vi "NI.History (EXT).vi"(1 "value in":ext) -> (0 "Stop?":bool)   [LabVIEW 2020]
doc: "Displays the value of the 32-bit signed integer numeric control and allows conditional breakpoints."
uses:
  <vilib>/Utility/miscctls.llb/LVRowAndColumnUnsignedTypeDef.ctl
panel:
  out "History":i32(listbox)=-1
  in  "Format":string="%#_g"
  in  "reset":bool
  # "* Changes to these options take effect the next time the probe runs."
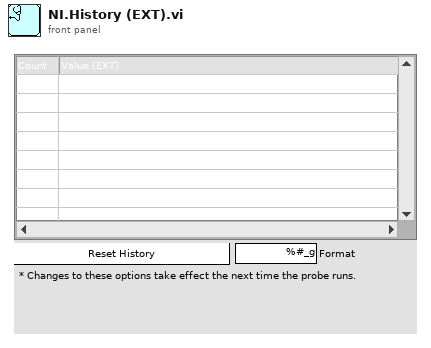
[diagram p1: front panel]
types:
  T1 = typedef "LVRowAndColumnUnsignedTypeDef.ctl" = cluster{"Row":u32, "Column":u32}
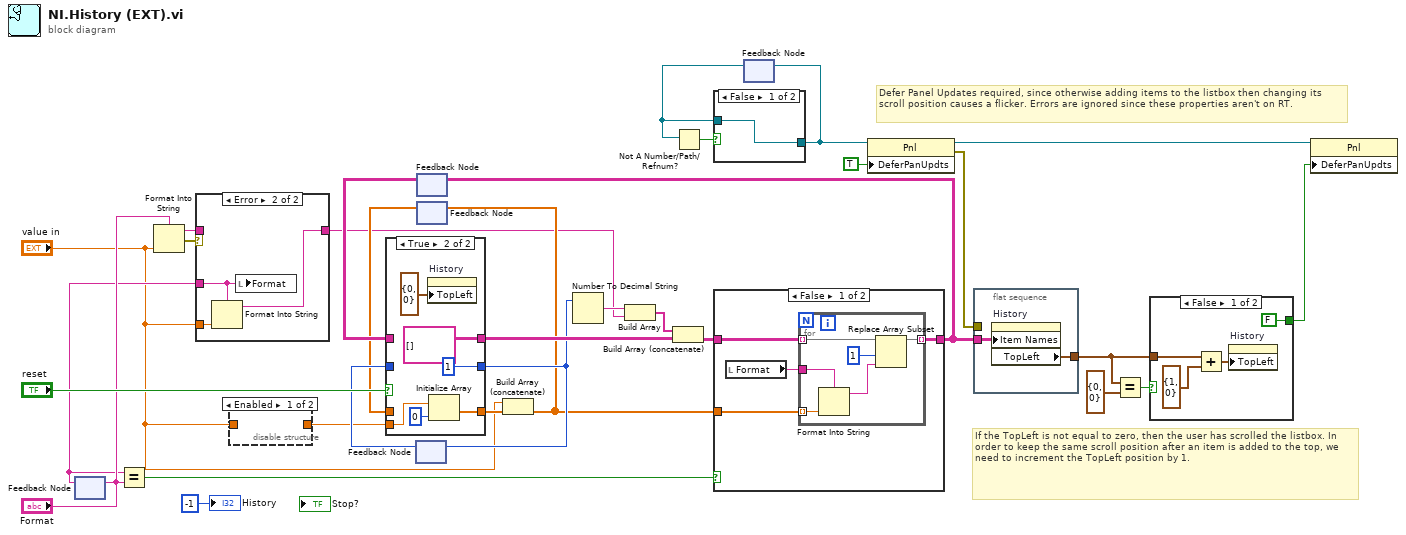
[diagram p0: block diagram]
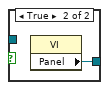
[diagram p3: hidden frame]
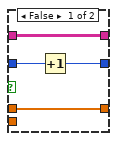
[diagram p6: hidden frame]
diagram:
  # "If the TopLeft is not equal to zero, then the user has scrolled the listbox. In order to keep the same scroll position after an item is added to the top, we need to increment the TopLeft position by 1."
  # "Defer Panel Updates required, since otherwise adding items to the listbox then changing its scroll position causes a flicker. Errors are ignored since these properties aren't on RT."
  n1 = feedback #1() -> (w15:string)  [unwired: 1 in]
  n2 = feedback-in #1("Format") -> ()
  n3 = Equal?(x=w15, y="Format") -> (x = y?=w17:bool)
  n4 = Format Into String(format string="Format", "value in") -> (resulting string=w12:string, error out=w13:errorcluster)  [unwired: 2 in]
  n5 = case shown="Error" w13 {
    tunnel: w15 -> [_ w34]
    tunnel: w12 -> [w32 _]
    tunnel: [w32 w33] -> w14
    tunnel: "value in" -> [_ w35]
    frame No Error {
    }
    frame Error {
      n6 = Format Into String(format string=w34, w35) -> (resulting string=w33:string)  [unwired: 2 in, 1 out]
      n7 = local write "Format"(w34) -> ()
    }
  }
  n8 = disable-structure shown="Enabled" {
    disable-tunnel: "value in" -> [_ w36]
    disable-tunnel: [_ w36] -> w21
    frame Enabled {
    }
    frame Disabled {
    }
  }
  n9 = feedback #2() -> (w25:i32)  [unwired: 1 in]
  n10 = feedback #3() -> (w24:string[][])  [unwired: 1 in]
  n11 = feedback #4() -> (w19:ext[])  [unwired: 1 in]
  n12 = case shown="True" "reset" {
    tunnel: w24 -> [w40 _]
    tunnel: w25 -> [w39 _]
    tunnel: [w40 string[][] []] -> w29
    tunnel: [w38 1] -> w26
    tunnel: w21 -> [_ w44]
    tunnel: [w37 w42] -> w20
    tunnel: w19 -> [w37 _]
    frame False {
      n13 = Increment(x=w39) -> (x+1=w38:i32)
    }
    frame True {
      n14 = property on="History" class="MCListbox (strict)"("TopLeft"=T1 {"Row"=0, "Column"=0} ("Top Left Visible Cell")) -> ()  [unwired: 2 in, 2 out]
      n15 = Initialize Array(w44, 0 ("dimension size")) -> (w42:ext[])
    }
  }
  n16 = feedback-in #2(w26) -> ()
  n17 = Build Array (concatenate)("value in", w20) -> (w18:ext[])
  n18 = feedback-in #4(w18) -> ()
  n19 = Number To Decimal String(number=w26) -> (decimal integer string=w27:string)  [unwired: 1 in]
  n20 = Build Array(w27, w14) -> (w28:string[])
  n21 = Build Array (concatenate)(w28, w29) -> (w22:string[][])
  n22 = case shown="False" w17 {
    tunnel: [w49 w57] -> w23
    tunnel: w22 -> [w50 w57]
    tunnel: w18 -> [w48 _]
    frame False {
      n23 = local read "Format"() -> (w47:string)
      n24 = for {
        tunnel: w50 -> [w56] mode=indexing
        tunnel: [w55] -> w49 mode=indexing
        tunnel: w48 -> [w53] mode=indexing
        tunnel: w47 -> [w51]
        n25 = Format Into String(format string=w51, w53) -> (resulting string=w52:string)  [unwired: 2 in, 1 out]
        n26 = Replace Array Subset(array=w56, new element=w52, index=1) -> (w55:string[])
      }
    }
    frame True {
    }
  }
  n27 = feedback-in #3(w23) -> ()
  n28 = feedback #5() -> (w7:refnum<vi>)  [unwired: 1 in]
  n29 = Not A Number/Path/Refnum?(number/path/refnum=w7) -> (NaN/Path/Refnum?=w8:bool)
  n30 = case shown="False" w8 {
    tunnel: [w58 w59] -> w9
    tunnel: w7 -> [w58 _]
    frame False {
    }
    frame True {
      n31 = property class="VI"() -> ("Panel"=w59:refnum<vi>)  [unwired: 2 in, 2 out]
    }
  }
  n32 = feedback-in #5(w9) -> ()
  n33 = property class="Pnl"(reference=w9, "DeferPanUpdts"=TRUE ("Defer Panel Updates")) -> (reference out=w6:refnum<vi>, error out=w5:errorcluster)  [unwired: 1 in]
  n34 = flat-sequence {
    tunnel: w23 -> [w61]
    tunnel: w5 -> [_]
    tunnel: [w60] -> w2
    frame #0 {
      n35 = property on="History" class="MCListbox (strict)"("Item Names"=w61) -> ("TopLeft"=w60:T1)  [unwired: 2 in, 2 out]
    }
  }
  n36 = Equal?(x=w2, y=T1 {"Row"=0, "Column"=0} ("Top Left Visible Cell")) -> (x = y?=w3:bool)
  n37 = case shown="False" w3 {
    tunnel: w2 -> [w65 _]
    tunnel: [FALSE ("Defer Panel Updates") _] -> w1
    frame False {
      n38 = Add(x=w65, y=T1 {"Row"=1, "Column"=0}) -> (x+y=w63:T1)
      n39 = property on="History" class="MCListbox (strict)"("TopLeft"=w63) -> ()  [unwired: 2 in, 2 out]
    }
    frame True {
    }
  }
  n40 = property class="Pnl"(reference=w6, "DeferPanUpdts"=w1) -> ()  [unwired: 1 in, 2 out]
  "History" <- -1 ("History of Values")
